vi "Temperature_Sensor_Calibration.vi"(11 "read__in":dbl format="%0.2f") -> (2 "Temperature":dbl, 3 "Temperature":dbl(knob) scale=0.0..100.0)   [LabVIEW 2022 SP3]
uses:
  <vilib>/ptbypt/NI_PtbyPt.lvlib
panel:
  out "mean":dbl format="%0.2f"
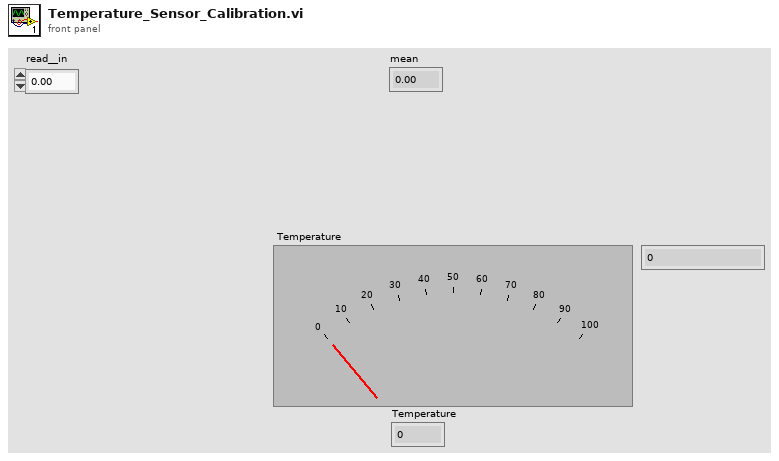
[diagram p1: front panel]
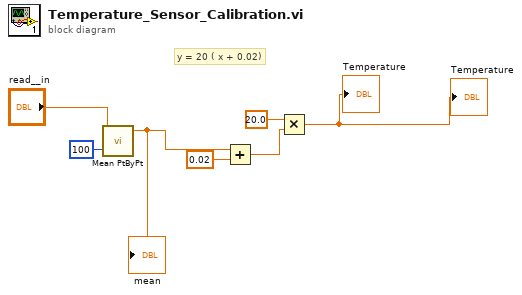
[diagram p0: block diagram]
diagram:
  # "y = 20 ( x + 0.02)"
  n1 = call <vilib>:"Mean PtByPt.vi"("x"="read__in", "sample length"=100) -> ("mean"=w5:dbl)  [unwired: 2 in, 1 out]
  "mean" <- w5
  n2 = Add(x=w5, y=0.02) -> (x+y=w4:dbl)
  n3 = Multiply(x=20.0, y=w4) -> (x*y=→"Temperature" →"Temperature":dbl)
